vi "FTW-Example-ActorConnector-Message.vi"() -> ()   [LabVIEW 2018]
uses:
  source/actor/Connector/FTW-ActorConnector.lvclass
  templates/Actor Template/Core/Actor Template-Core.lvclass
  source/actor/Ether/FTW-Ether.lvclass
panel:
  in  "Ping":bool
  out "Instance Inbox Address":string
  out "Initialized Response":string
  out "Timed out?":bool
  out "Ping Response":string
  in  "FTW Ether Configuration":string="{\n  \"ApplicationName\": \"Actor Connector Example\",\n  \"ApplicationVersion\": \"0.1.0-1\",\n  \"LoggerAddress\": \"inproc://*\",\n  \"LoggerName\": \"ActorConnectorExample\",\n  \"LoggerDirectory\": \"[UserDesktop]\\\\Logs\",\n  \"LoggerDiskThrashDelay\": 200\n}"
  in  "Actor 1 Configuration":string="{\n  \"Identity\": \"FeatherweightActorConnectorExample\",\n  \"InboxAddress\": \"inproc://*\",\n  \"LoggerAddress\": \"\",\n  \"DebugEnableInboxLogging\": false,\n  \"DebugEnableJobLogging\": false,\n  \"DebugShowPanel\": false\n}"
  out "error out":errorcluster
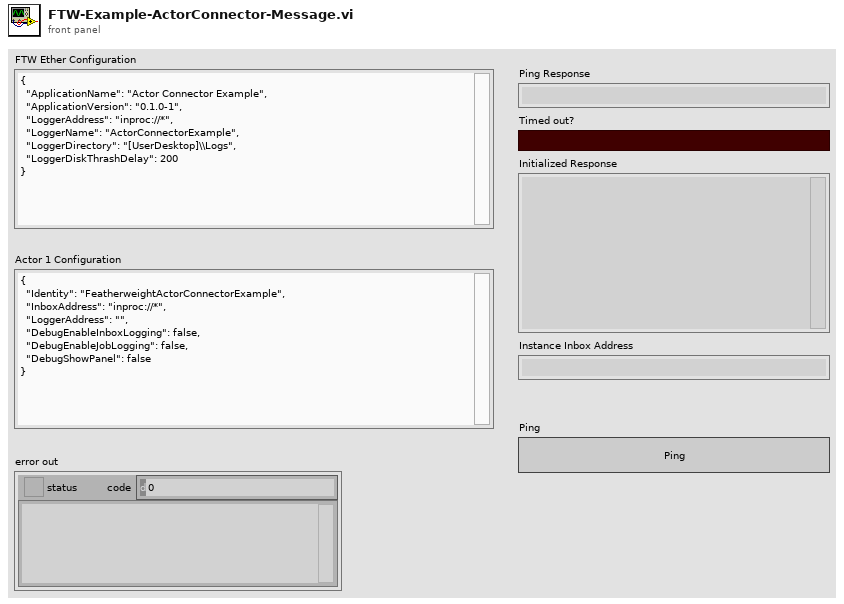
[diagram p1: front panel]
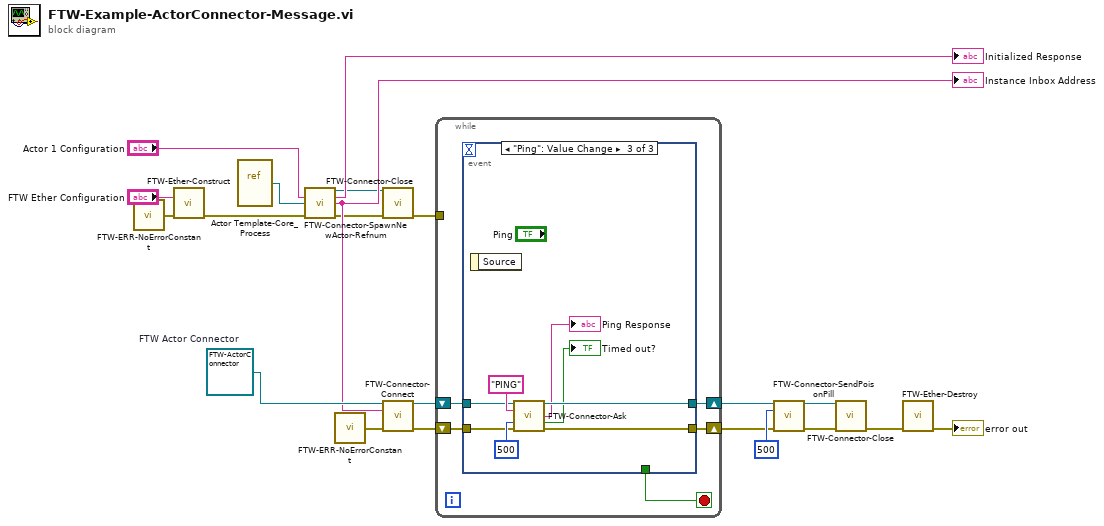
[diagram p0: block diagram]
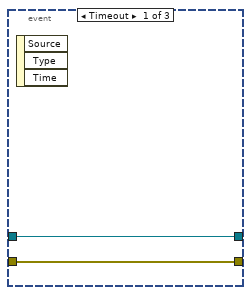
[diagram p2: hidden frame]
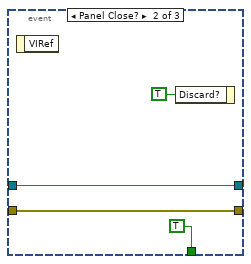
[diagram p3: hidden frame]
diagram:
  w13 = refnum<class "FTW-ActorConnector.lvclass"> refnum  # FTW Actor Connector
  n1 = call "FTW-ERR-NoErrorConstant.vi"() -> ("no error"=w11:errorcluster)
  n2 = call "FTW-Ether-Construct.vi"("FTW Ether Configuration"="FTW Ether Configuration", "error in"=w11) -> ("error out"=w21:errorcluster)  [unwired: 13 in]
  n3 = vi-ref "Actor Template-Core_Process.vi"() -> (w1:refnum<vi>)
  n4 = call "FTW-Connector-SpawnNewActor-Refnum.vi"("Configuration"="Actor 1 Configuration", "Actor VI Refnum"=w1, "error in"=w21) -> ("FTW Actor Connector"=w8:refnum<class "FTW-ActorConnector.lvclass">, "Initialized Response"=→"Initialized Response":string, "Instance Inbox Address"=w12:string, "error out"=w9:errorcluster)  [unwired: 9 in]
  "Instance Inbox Address" <- w12
  n5 = call "FTW-ERR-NoErrorConstant.vi"() -> ("no error"=w10:errorcluster)
  n6 = call-dynamic "FTW-Connector-Close.vi"("FTW Actor Connector"=w8, "error in"=w9) -> ("error out"=w5:errorcluster)  [unwired: 13 in]
  n7 = call-dynamic "FTW-Connector-Connect.vi"("FTW Actor Connector Type"=w13, "Instance Inbox Address"=w12, "error in"=w10) -> ("FTW Actor Connector"=w6:refnum<class "FTW-ActorConnector.lvclass">, "error out"=w7:errorcluster)  [unwired: 11 in]
  n8 = while {
    shift-right: [w23] -> w3
    shift-left: w6 -> [w24]
    shift-right: [w22] -> w4
    shift-left: w7 -> [w25]
    tunnel: w5 -> [_]
    stop <- w26 stop-if-true
    n9 = event shown="[2] \"Ping\": Value Change" {
      selector: _ -> [_ _ _]
      dyn-events: _ -> [_ _ _]
      timeout: _ -> [_ _ _]
      tunnel: [_ TRUE _] -> w26
      tunnel: w25 -> [w28 w30 w38]
      tunnel: [w28 w30 w37] -> w22
      tunnel: w24 -> [w27 w29 w36]
      tunnel: [w27 w29 w35] -> w23
      event Timeout {
        n10 = event-data() -> ()  [unwired: 1 in, 3 out]
      }
      event Panel Close? {
        n11 = event-data() -> ()  [unwired: 1 in, 1 out]
        n12 = event-data("Discard?"=TRUE) -> ()  [unwired: 1 in, 1 out]
      }
      event "Ping": Value Change {
        n13 = event-data() -> ()  [unwired: 1 in, 1 out]
        n14 = call "FTW-Connector-Ask.vi"("FTW Actor Connector"=w36, "Request Header"="PING", "Timeout"=500, "error in"=w38) -> ("FTW Actor Connector out"=w35:refnum<class "FTW-ActorConnector.lvclass">, "Response Body"=→"Ping Response":string, "Timed out?"=→"Timed out?":bool, "error out"=w37:errorcluster)  [unwired: 6 in, 2 out]
      }
    }
  }
  n15 = call-dynamic "FTW-Connector-SendPoisonPill.vi"("FTW Actor Connector"=w3, "Timeout"=500, "error in"=w4) -> ("FTW Actor Connector out"=w16:refnum<class "FTW-ActorConnector.lvclass">, "error out"=w15:errorcluster)  [unwired: 7 in, 4 out]
  n16 = call-dynamic "FTW-Connector-Close.vi"("FTW Actor Connector"=w16, "error in"=w15) -> ("error out"=w18:errorcluster)  [unwired: 13 in]
  n17 = call "FTW-Ether-Destroy.vi"("error in"=w18) -> ("error out"=→"error out":errorcluster)  [unwired: 14 in]
